vi "GPS Weather Sub VI.vi"(0 "VISA resource name out":refnum<visa-resource-name>, 5 "error out":errorcluster) -> (9 "Weather":string, 10 "Latitude":string, 11 "Altitude":string, 12 "Longitude":string, 13 "# of satellites":string, 14 "VISA resource name out 2":refnum<visa-resource-name>, 15 "Time":string, 16 "Base speed (mph)":dbl, 17 "Base Heading (degrees)":dbl, 18 "Date":string, 19 "error IO":errorcluster)   [LabVIEW 2009]
doc: "This subVI decodes the most common NMEA-0183 sentence transmitted by GPS receivers, the $GPRMC sentence. The subvi returns time, position, ground speed, and magnetic variation. In the GPS interface configuration, use the \"NMEA OUT\" setting and set the baud rate to the standard 4800 bps setting. Connected to the computer's serial port using a PC Interface Cable, available from the GPS vendor. This subvi initializes the serial port on first call. On subsequent calls, the initialization is skipped. Always use the Stop input when stopping the VI so that the serial port connection is closed."
uses:
  <vilib>/regexp/Match Regular Expression.xnode
panel:
  out "concatenated string 2":string
  out "read buffer":string
  out "before match":string
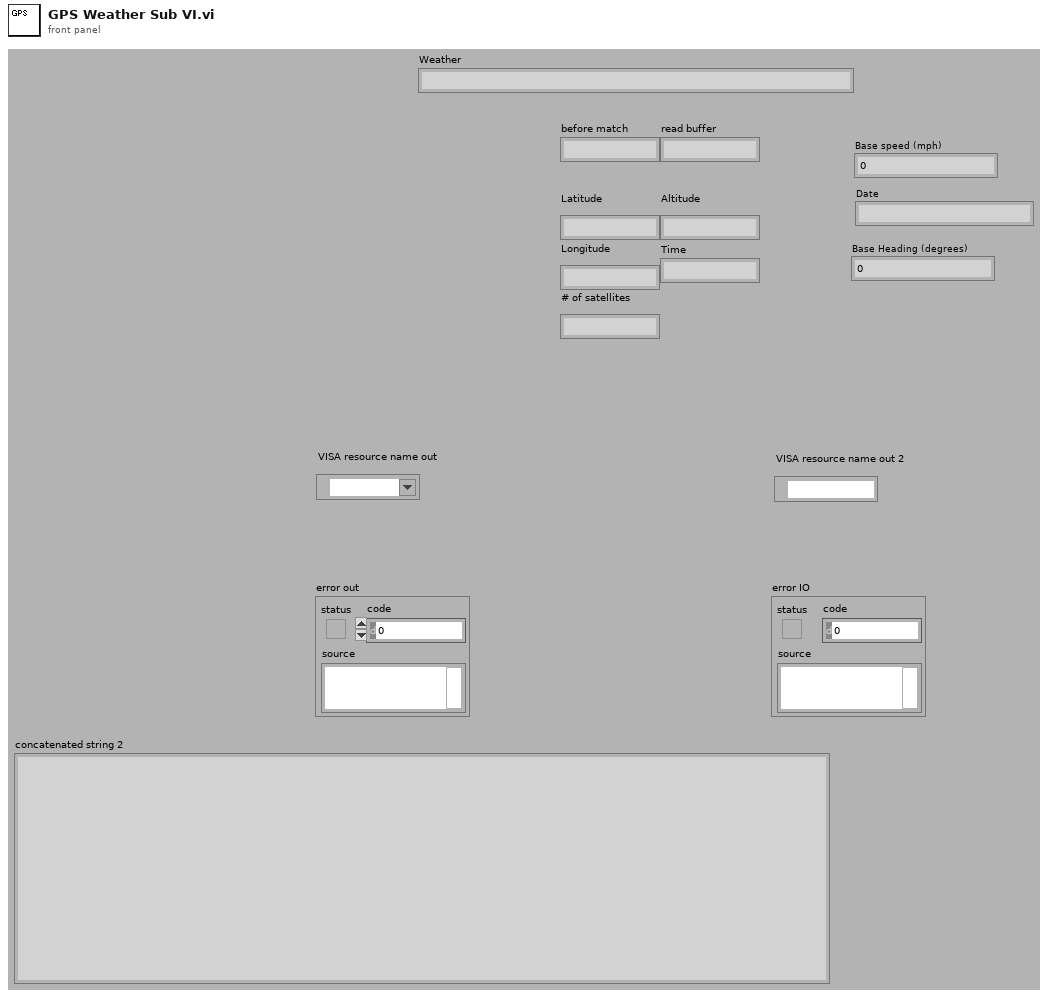
[diagram p1: front panel]
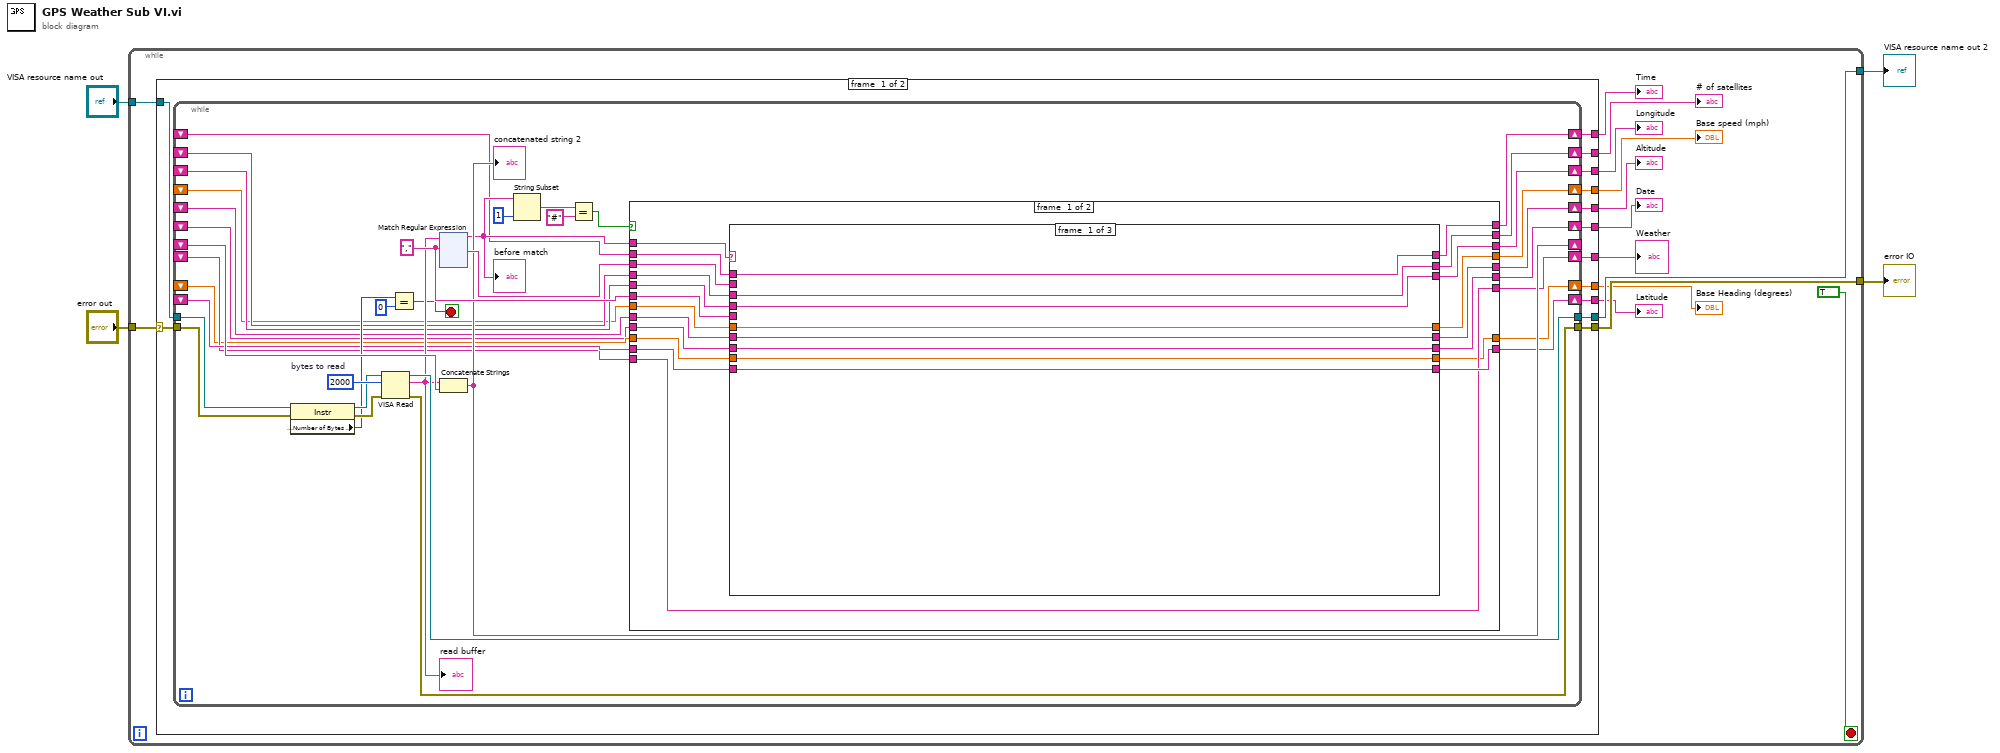
[diagram p0: block diagram]
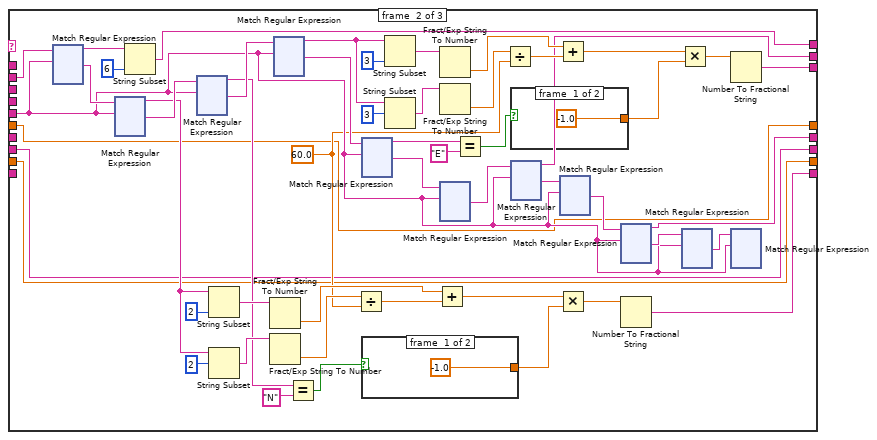
[diagram p2: hidden frame]
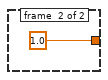
[diagram p3: hidden frame]
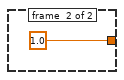
[diagram p4: hidden frame]
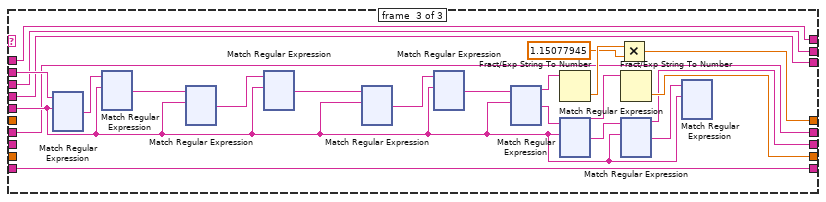
[diagram p5: hidden frame]
diagram:
  n1 = while {
    tunnel: "VISA resource name out" -> [w18]
    tunnel: "error out" -> [w17]
    tunnel: [w16] -> w2
    tunnel: [w14] -> w1
    stop <- TRUE stop-if-true
    n2 = case shown="No Error" w17 {
      selector: w17 -> [w30 w2539]
      tunnel: w18 -> [w31 w2540]
      tunnel: [w29 w2540] -> w14
      tunnel: [w28 w2539] -> w16
      tunnel: [w27 _] -> w13
      tunnel: [w26 _] -> w12
      tunnel: [w25 _] -> w11
      tunnel: [w24 _] -> w10
      tunnel: [w23 _] -> w9
      tunnel: [w22 _] -> w8
      tunnel: [w21 _] -> w7
      tunnel: [w20 _] -> w6
      tunnel: [w19 _] -> w5
      frame #0 {
        n3 = while {
          tunnel: w31 -> [w60]
          tunnel: w30 -> [w61]
          tunnel: [w66] -> w29
          tunnel: [w65] -> w28
          shift-right: [w63] -> _
          shift-left: _ -> [w64]
          shift-right: [w49] -> w27
          shift-left: _ -> [w48]
          shift-right: [w47] -> w26
          shift-left: _ -> [w46]
          shift-right: [w45] -> w25
          shift-left: _ -> [w44]
          shift-right: [w43] -> w24
          shift-left: _ -> [w42]
          shift-right: [w41] -> w23
          shift-left: _ -> [w40]
          shift-right: [w39] -> w22
          shift-left: _ -> [w38]
          shift-right: [w37] -> w21
          shift-left: _ -> [w36]
          shift-right: [w35] -> w20
          shift-left: _ -> [w34]
          shift-right: [w33] -> w19
          shift-left: _ -> [w32]
          stop <- w56 stop-if-true
          w67 = "," ("regular expression")
          w69 = u32 2000  # bytes to read
          n4 = property class="Instr"(reference=w60, error in=w61) -> (reference out=w59:refnum<visa-resource-name>, error out=w58:errorcluster, "Serial Settings:Number of Bytes at Serial Port"=w55:u32)
          n5 = VISA Read(VISA resource name=w59, byte count=w69, error in (no error)=w58) -> (VISA resource name out=w66:refnum<visa-resource-name>, read buffer=w62:string, error out=w65:errorcluster)  [unwired: 1 out]
          "read buffer" <- w62
          n6 = Equal?(x=w55, y=u32 0) -> (x = y?=w56:bool)
          n7 = xnode "Match Regular Expression"("input string"=w62, "regular expression"=w67) -> ("before match"=w53:string, "after match"=w68:string)  [unwired: 2 in, 5 out]
          "before match" <- w53
          n8 = Concatenate Strings(w62, w64) -> (w63:string)
          "concatenated string 2" <- w63
          n9 = String Subset(string=w53, length (rest)=1 ("length (rest)")) -> (substring=w51:string)  [unwired: 1 in]
          n10 = Equal?(x=w51, y="#") -> (x = y?=w50:bool)
          n11 = case shown="False" w50 {
            tunnel: w68 -> [w89 w2430]
            tunnel: w67 -> [w88 _]
            tunnel: w53 -> [w87 _]
            tunnel: [w86 w2431] -> w49
            tunnel: w48 -> [w85 w2431]
            tunnel: [w84 w2430] -> w47
            tunnel: w46 -> [w84 _]
            tunnel: [w83 w2429] -> w45
            tunnel: w44 -> [w82 w2429]
            tunnel: [w81 w2428] -> w43
            tunnel: w42 -> [w80 w2428]
            tunnel: [w79 w2427] -> w41
            tunnel: w40 -> [w78 w2427]
            tunnel: [w77 w2426] -> w39
            tunnel: w38 -> [w76 w2426]
            tunnel: [w75 w2425] -> w37
            tunnel: w36 -> [w74 w2425]
            tunnel: [w73 w2424] -> w35
            tunnel: w34 -> [w72 w2424]
            tunnel: [w71 w2423] -> w33
            tunnel: w32 -> [w70 w2423]
            frame #0 {
              n12 = case shown="\"$GPGGA\"" w87 {
                tunnel: w89 -> [_ w148 w1340]
                tunnel: w88 -> [_ w137 w1341]
                tunnel: [w97 w105 w1337] -> w86
                tunnel: w85 -> [w97 _ w1337]
                tunnel: [w96 w104 w1336] -> w83
                tunnel: w82 -> [w96 _ w1336]
                tunnel: [w95 w103 w1335] -> w81
                tunnel: w80 -> [w95 _ w1335]
                tunnel: [w94 w98 w1334] -> w79
                tunnel: w78 -> [w94 _ w1334]
                tunnel: [w93 w102 w1333] -> w77
                tunnel: w76 -> [w93 _ w1333]
                tunnel: [w92 w101 w1332] -> w75
                tunnel: w74 -> [w92 w101 _]
                tunnel: [w91 w100 w1331] -> w73
                tunnel: w72 -> [w91 w100 _]
                tunnel: [w90 w99 w1330] -> w71
                tunnel: w70 -> [w90 w99 _]
                frame #0 {
                }
                frame #1 {
                  w120 = 60.0 ("y")
                  n13 = xnode "Match Regular Expression"("input string"=w148, "regular expression"=w137) -> ("before match"=w106:string, "after match"=w147:string)  [unwired: 2 in, 5 out]
                  n14 = xnode "Match Regular Expression"("input string"=w147, "regular expression"=w137) -> ("before match"=w129:string, "after match"=w146:string)  [unwired: 2 in, 5 out]
                  n15 = String Subset(string=w106, length (rest)=6 ("length (rest)")) -> (substring=w103:string)  [unwired: 1 in]
                  n16 = xnode "Match Regular Expression"("input string"=w146, "regular expression"=w137) -> ("before match"=w119:string, "after match"=w145:string)  [unwired: 2 in, 5 out]
                  n17 = String Subset(string=w129, length (rest)=2 ("length (rest)")) -> (substring=w132:string)  [unwired: 1 out]
                  n18 = String Subset(string=w129, offset (0)=2) -> (substring=w134:string)  [unwired: 1 out]
                  n19 = Fract/Exp String To Number(string=w132) -> (number=w131:dbl)  [unwired: 4 out]
                  n20 = Fract/Exp String To Number(string=w134) -> (number=w133:dbl)  [unwired: 4 out]
                  n21 = xnode "Match Regular Expression"("input string"=w145, "regular expression"=w137) -> ("before match"=w121:string, "after match"=w144:string)  [unwired: 2 in, 5 out]
                  n22 = Equal?(x=w119, y="N") -> (x = y?=w117:bool)
                  n23 = Divide(x=w133, y=w120) -> (x/y=w130:dbl)
                  n24 = xnode "Match Regular Expression"("input string"=w144, "regular expression"=w137) -> ("before match"=w112:string, "after match"=w143:string)  [unwired: 2 in, 5 out]
                  n25 = case shown="False" w117 {
                    tunnel: [-1.0 ("y") 1.0 ("y")] -> w115
                    frame #0 {
                    }
                    frame #1 {
                    }
                  }
                  n26 = String Subset(string=w121, length (rest)=3 ("length (rest)")) -> (substring=w126:string)  [unwired: 1 out]
                  n27 = String Subset(string=w121, offset (0)=3) -> (substring=w128:string)  [unwired: 1 out]
                  n28 = Add(x=w131, y=w130) -> (x+y=w116:dbl)
                  n29 = Fract/Exp String To Number(string=w126) -> (number=w125:dbl)  [unwired: 4 out]
                  n30 = Fract/Exp String To Number(string=w128) -> (number=w127:dbl)  [unwired: 4 out]
                  n31 = xnode "Match Regular Expression"("input string"=w143, "regular expression"=w137) -> ("after match"=w142:string)  [unwired: 2 in, 6 out]
                  n32 = Equal?(x=w112, y="E") -> (x = y?=w111:bool)
                  n33 = Divide(x=w127, y=w120) -> (x/y=w124:dbl)
                  n34 = case shown="False" w111 {
                    tunnel: [-1.0 ("y") 1.0 ("y")] -> w109
                    frame #0 {
                    }
                    frame #1 {
                    }
                  }
                  n35 = xnode "Match Regular Expression"("input string"=w142, "regular expression"=w137) -> ("before match"=w98:string, "after match"=w141:string)  [unwired: 2 in, 5 out]
                  n36 = Add(x=w125, y=w124) -> (x+y=w110:dbl)
                  n37 = Multiply(x=w116, y=w115) -> (x*y=w114:dbl)
                  n38 = xnode "Match Regular Expression"("input string"=w141, "regular expression"=w137) -> ("after match"=w140:string)  [unwired: 2 in, 6 out]
                  n39 = xnode "Match Regular Expression"("input string"=w140, "regular expression"=w137) -> ("before match"=w102:string, "after match"=w139:string)  [unwired: 2 in, 5 out]
                  n40 = Number To Fractional String(number=w114) -> (F-format string=w105:string)  [unwired: 3 out]
                  n41 = Multiply(x=w110, y=w109) -> (x*y=w108:dbl)
                  n42 = xnode "Match Regular Expression"("input string"=w139, "regular expression"=w137) -> ("after match"=w138:string)  [unwired: 2 in, 6 out]
                  n43 = Number To Fractional String(number=w108) -> (F-format string=w104:string)  [unwired: 3 out]
                  n44 = xnode "Match Regular Expression"("input string"=w138, "regular expression"=w137) -> ()  [unwired: 2 in, 7 out]
                }
                frame #2 {
                  n45 = xnode "Match Regular Expression"("input string"=w1340, "regular expression"=w1341) -> ("after match"=w1352:string)  [unwired: 2 in, 6 out]
                  n46 = xnode "Match Regular Expression"("input string"=w1352, "regular expression"=w1341) -> ("after match"=w1351:string)  [unwired: 2 in, 6 out]
                  n47 = xnode "Match Regular Expression"("input string"=w1351, "regular expression"=w1341) -> ("after match"=w1350:string)  [unwired: 2 in, 6 out]
                  n48 = xnode "Match Regular Expression"("input string"=w1350, "regular expression"=w1341) -> ("after match"=w1345:string)  [unwired: 2 in, 6 out]
                  n49 = xnode "Match Regular Expression"("input string"=w1345, "regular expression"=w1341) -> ("after match"=w1349:string)  [unwired: 2 in, 6 out]
                  n50 = xnode "Match Regular Expression"("input string"=w1349, "regular expression"=w1341) -> ("after match"=w1348:string)  [unwired: 2 in, 6 out]
                  n51 = xnode "Match Regular Expression"("input string"=w1348, "regular expression"=w1341) -> ("before match"=w1339:string, "after match"=w1347:string)  [unwired: 2 in, 5 out]
                  n52 = Fract/Exp String To Number(string=w1339) -> (number=w1343:dbl)  [unwired: 4 out]
                  n53 = xnode "Match Regular Expression"("input string"=w1347, "regular expression"=w1341) -> ("before match"=w1338:string, "after match"=w1346:string)  [unwired: 2 in, 5 out]
                  n54 = Multiply(x=w1343, y=1.15077945) -> (x*y=w1332:dbl)
                  n55 = Fract/Exp String To Number(string=w1338) -> (number=w1331:dbl)  [unwired: 4 out]
                  n56 = xnode "Match Regular Expression"("input string"=w1346, "regular expression"=w1341) -> ("before match"=w1330:string, "after match"=w1344:string)  [unwired: 2 in, 5 out]
                  n57 = xnode "Match Regular Expression"("input string"=w1344, "regular expression"=w1341) -> ()  [unwired: 2 in, 7 out]
                }
              }
            }
            frame #1 {
            }
          }
        }
      }
      frame #1 {
      }
    }
    "Latitude" <- w13
    "Weather" <- w12
    "Longitude" <- w11
    "Time" <- w10
    "# of satellites" <- w9
    "Altitude" <- w8
    "Base speed (mph)" <- w7
    "Base Heading (degrees)" <- w6
    "Date" <- w5
  }
  "error IO" <- w2
  "VISA resource name out 2" <- w1
